vi "HighPassFilterST.vi"(8 "init/cont (init:F)":bool, 10 "Doppler Params":T1={"Dopp Filter Order"=2, "Window length"=64, "Window Increment"=64, "Start f"=0.05, "lDoppler cutouff"=10.0, "FFT Length"=512, "SlowTime (Hz)"=100.0} {"Start f" format="%0.3f"; "SlowTime (Hz)" format="%0.1f"; "lDoppler cutouff" format="%0.3f"}, 11 "slow time":csg[](array[numeric])) -> (2 "Filtered X":csg[](array[numeric]), 5 "Slow time sampling":dbl, 6 "error":i32)   [LabVIEW 2022 SP3]
uses:
  DopplerParams.ctl
  <vilib>/Analysis/3filter.llb/Butterworth Filter (CDB).vi
  <vilib>/Analysis/3filter.llb/Equi-Ripple HighPass (CDB).vi
  <vilib>/Analysis/3filter.llb/Filter Passband Type.ctl
  <vilib>/Analysis/NI_AALBase.lvlib
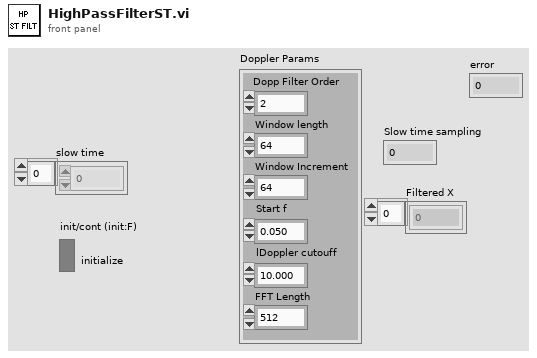
[diagram p1: front panel]
types:
  T1 = typedef "DopplerParams.ctl" = cluster{"Dopp Filter Order":i32, "Window length":i32, "Window Increment":i32, "Start f":dbl, "lDoppler cutouff":dbl, "FFT Length":i32, "SlowTime (Hz)":dbl}
  T2 = typedef "NI_AALBase.lvlib/Filter Passband Type.ctl" = enum32{"Lowpass", "Highpass", "Bandpass", "Bandstop"}
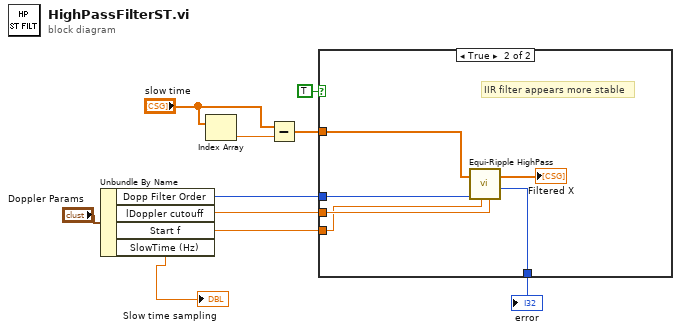
[diagram p0: block diagram]
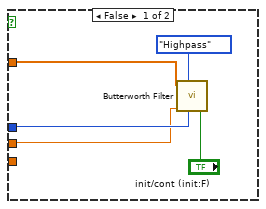
[diagram p2: hidden frame]
diagram:
  n1 = Unbundle By Name("Doppler Params") -> ("Dopp Filter Order"=w7:i32, "lDoppler cutouff"=w1:dbl, "Start f"=w2:dbl, "SlowTime (Hz)"=→"Slow time sampling":dbl)
  n2 = Index Array(array="slow time") -> (element=w9:csg)  [unwired: 1 in]
  n3 = Subtract(x="slow time", y=w9) -> (x-y=w8:csg[])
  n4 = case shown="True" TRUE {
    tunnel: w8 -> [w15 w21]
    tunnel: w7 -> [w13 w20]
    tunnel: w1 -> [w11 w17]
    tunnel: w2 -> [_ w16]
    tunnel: [_ w18] -> w3
    frame False {
      n5 = call-poly <vilib>:"Butterworth Filter.vi"("init/cont (init:F)"="init/cont (init:F)", "order"=w13, "filter type"=Filter_Passband_Type."Highpass", "low cutoff freq: fl"=w11, "X"=w15) -> ()  [unwired: 3 in, 2 out]
    }
    frame True {
      # "IIR filter appears more stable"
      n6 = call-poly <vilib>:"Equi-Ripple HighPass.vi"("# of taps"=w20, "stop freq"=w16, "high freq"=w17, "X"=w21) -> ("error"=w18:i32, "Filtered X"=→"Filtered X":cdb[])  [unwired: 2 in]
    }
  }
  "error" <- w3
